vi "MDOAcquire Data from х502 streaming.vi"() -> ()   [LabVIEW 2012]
uses:
  controls/Coeff.ctl
  controls/MDOHW Configuration.ctl
  <vilib>/Analysis/3filter.llb/Filter Passband Type.ctl
  <vilib>/Analysis/3filter.llb/Butterworth Filter (DBL).vi
  <vilib>/Analysis/NI_AALBase.lvlib
panel:
  in  "Hardware Configuration":T1 {"SyncMode" items=["INTERNAL"=0, "EXTERNAL_MASTER"=1, "DI_SYN1_RISE"=2, "DI_SYN1_FALL"=3, "DI_SYN2_RISE"=6, "DI_SYN2_FALL"=7]}
  in  "Coeff":T2={"Coeff_U"=300.0, "Offset_U"=0.0, "Coeff_I"=23.5, "Offset_I"=0.15}
  in  "stop":bool
  out "error out":errorcluster
  in  "error in (no error)":errorcluster
  out "din_data_size":u32
  out "Ток":dbl[](graph)
  out "Напряжение":dbl[](graph)
  out "DIN":u32[](array[numeric]) format="%b"
  in  "IP Addr":string="192.168.0.1"
  out "MCU ver":string
  in  "Отображать за время":dbl=100.0 min=10.0 step=1.0
  out "Установленная частота синхронного ввода DIN":dbl=2.0 min=2.0 max=2000000.0 format="%#_8f"
  in  "Частота синхронного ввода DIN":dbl=20000.0 min=1.0 max=2000000.0 format="%#_8f"
  out "FPGA Ver":string
  out "Установленная частота на канал":dbl=2.0 min=2.0 max=2000000.0 format="%#_8f"
  out "Установленная частота сбора":dbl=2.0 min=2.0 max=2000000.0 format="%#_8f"
  in  "Частота сбора на канал":dbl=50000.0 min=2.0 max=2000000.0 format="%#_8f"
  in  "Частота сбора (Гц)":dbl=100000.0 min=2.0 max=2000000.0 format="%#_8f"
  out "PldaVer":u8
  out "Serial":string
  out "Name":string
  # "Информация о плате"
  # "Настройки модуля"
  # "Устанавливаемое"
  # "Установленное"
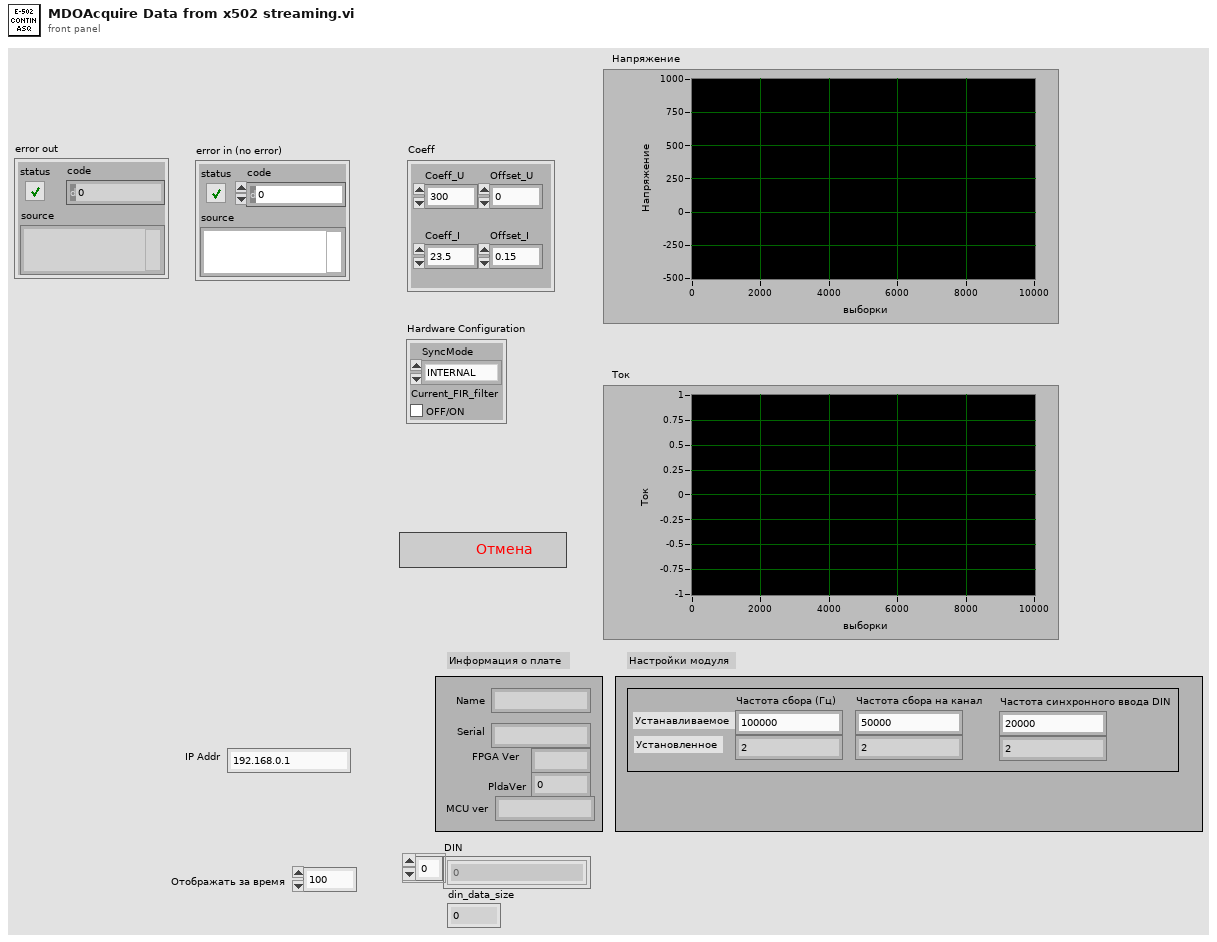
[diagram p1: front panel]
types:
  T1 = typedef "MDOHW Configuration.ctl" = cluster{"SyncMode":u32, "Current_FIR_filter":bool}
  T2 = typedef "Coeff.ctl" = cluster{"Coeff_U":dbl, "Offset_U":dbl, "Coeff_I":dbl, "Offset_I":dbl}
  T3 = cluster{"PhyCh":u32, "Avg":u32, "Mode":u32, "Range":u32}[]
  T4 = typedef "NI_AALBase.lvlib/Filter Passband Type.ctl" = enum32{"Lowpass", "Highpass", "Bandpass", "Bandstop"}
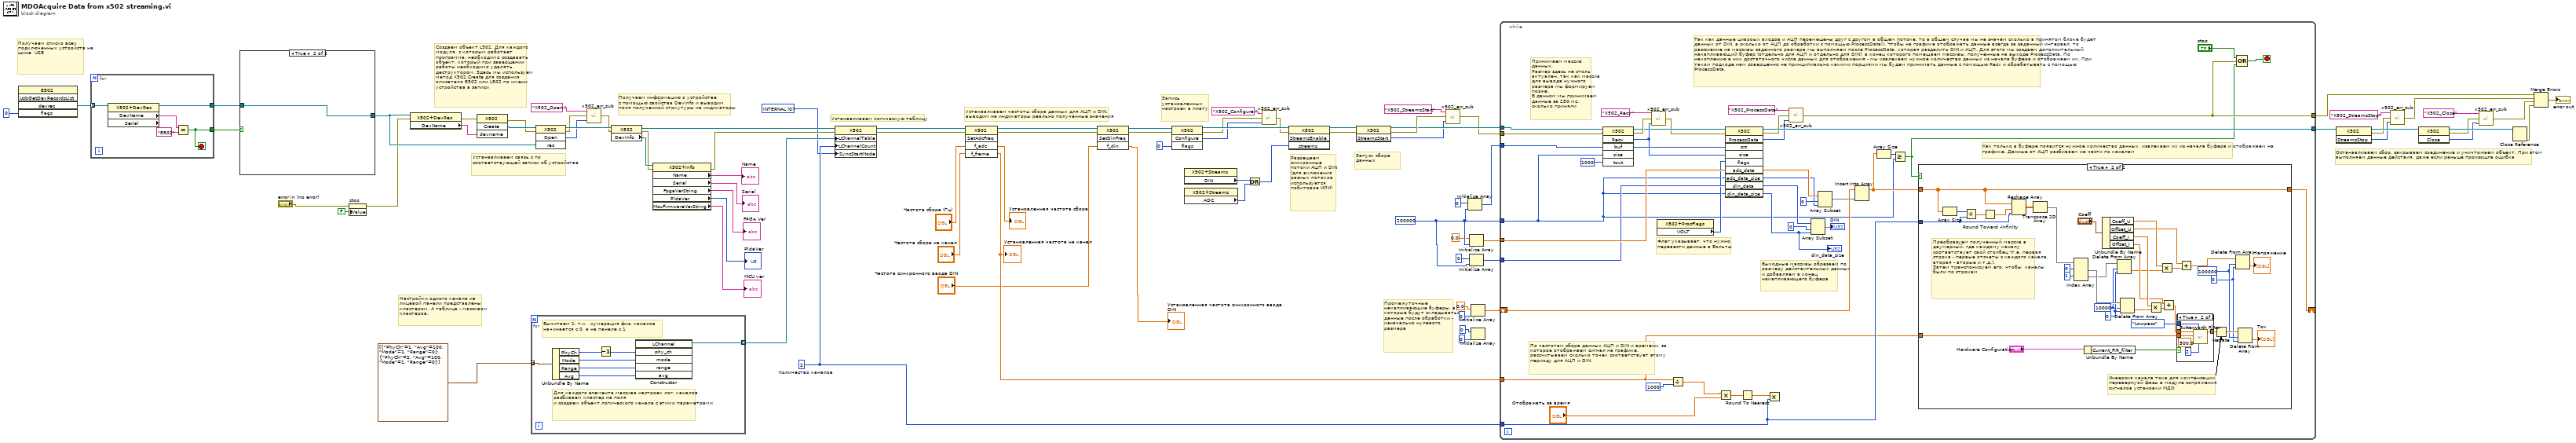
[diagram p0: block diagram]
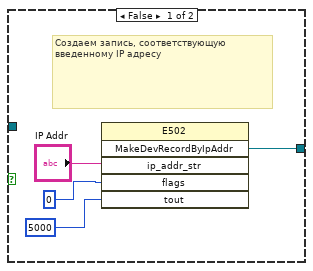
[diagram p4: hidden frame]
diagram:
  w1 = u32 0 items=["INTERNAL"=0, "EXTERNAL_MASTER"=1, "DI_SYN1_RISE"=2, "DI_SYN1_FALL"=3, "DI_SYN2_RISE"=6, "DI_SYN2_FALL"=7] ("SyncStartMode")
  w84 = u32 2  # Количество каналов
  w80 = u32 200000 ("element")
  # "Промежуточные накапливающие буферы, в которые будут складываться данные после обработки - изначально нулевого размера"
  # "Получаем списко всех подключенных устройств на шине  USB"
  # "Останавливаем сбор, закрываем соединение и уничтожаем объект. При этом выполняем данные действия, даже если раньше произошла ошибка"
  # "Запуск сбора данных"
  # "Разрешаем синхронные потоки АЦП и DIN (для включения разных потоков используется побитовое ИЛИ)"
  # "Запись установленных настроек в плату"
  # "Устанавливаем частоты сбора данных для АЦП и DIN,\nвыводим на индикаторы реально полученные значения"
  # "Устанавливаем логическую таблицу"
  # "Настройки одного канала на лицевой панели представлены кластером. А таблица - массивом кластеров."
  # "Создаем объект L502. Для каждого модуля, с которым работает программа, необходимо создавать объект, который при завершении работы необходимо удалять деструктором. Здесь мы используем метод X502.Create для создания описателя E502 или L502 по имени устройства в записи"
  # "Получаем информацию о устройстве \nс помощью свойства DevInfo и выводим\nполя полученной стркутуры на индикаторы"
  # "Устанавливаем связь с по соответствующей записи об устройстве"
  n1 = invoke class="E502" method="UsbGetDevRecordsList"("flags"=0) -> ("devrec"=w14:refnum<k24>[])  [unwired: 4 in, 4 out]
  n2 = for {
    tunnel: w14 -> [w89] mode=indexing
    tunnel: [w88] -> w12
    tunnel: [w85] -> w13
    stop <- w85 stop-if-true
    n3 = property class="X502+DevRec" props=["DevName", "Serial"](reference=w89) -> (reference out=w88:refnum<k24>, "DevName"=w87:string)  [unwired: 1 in, 2 out]
    n4 = Equal?(x=w87, y="E502") -> (x = y?=w85:bool)
  }
  n5 = case shown="True" w13 {
    tunnel: [w90 w94] -> w21
    tunnel: w12 -> [_ w94]
    frame False {
      # "Создаем запись, соответствующую введенному IP адресу"
      n6 = invoke class="E502" method="MakeDevRecordByIpAddr"("ip_addr_str"="IP Addr", "flags"=0, "tout"=5000) -> ("MakeDevRecordByIpAddr"=w90:refnum<k24>)  [unwired: 3 in, 5 out]
    }
    frame True {
    }
  }
  n7 = property on="stop" class="Bool (strict)"(error in="error in (no error)", "Value"=FALSE ("Visible")) -> (error out=w9:errorcluster)  [unwired: 1 in, 1 out]
  n8 = property class="X502+DevRec"(reference=w21, error in=w9) -> (error out=w16:errorcluster, "DevName"=w52:string)  [unwired: 1 out]
  n9 = invoke class="X502" method="Create"(error in=w16, "devname"=w52) -> (error out=w51:errorcluster, "Create"=w53:refnum<k24>)  [unwired: 2 in, 2 out]
  n10 = for {
    tunnel: T3 [{"PhyCh"=1, "Avg"=100, "Mode"=1, "Range"=0}, {"PhyCh"=2, "Avg"=100, "Mode"=1, "Range"=0}] ("Логические каналы") -> [w101] mode=indexing
    tunnel: [w95] -> w76 mode=indexing
    # "Вычитаем 1, т.к.  нумерация физ. каналов начинается с 0, а на панеле с 1"
    # "Для каждого элемента массива настроек лог. каналов разбиваем кластер на поля\nи создаем объект логического канала с этими параметрами"
    n11 = Unbundle By Name(w101) -> ("PhyCh"=w100:u32, "Mode"=w98:u32, "Range"=w97:u32, "Avg"=w96:u32)
    n12 = Decrement(x=w100) -> (x-1=w99:u32)
    n13 = constructor class="X502+LChannel"("phy_ch"=w99, "mode"=w98, "range"=w97, "avg"=w96) -> (reference out=w95:refnum<k24>)  [unwired: 3 in, 6 out]
  }
  n14 = invoke class="X502" method="Open"(reference=w53, error in=w51, "rec"=w21) -> (reference out=w56:refnum<k24>, error out=w49:errorcluster, "Open"=w50:i32)  [unwired: 1 in, 1 out]
  n15 = call "x502_err_sub.vi"("Error code"=w50, "error in (no error)"=w49, "Error descr"="X502_Open ") -> ("error out"=w47:errorcluster)
  n16 = property class="X502"(reference=w56, error in=w47) -> (reference out=w57:refnum<k24>, error out=w45:errorcluster, "DevInfo"=w46:refnum<k24>)
  n17 = property class="X502+Info"(reference=w46, error in=w45) -> (error out=w22:errorcluster, "Name"=→"Name":string, "Serial"=→"Serial":string, "FpgaVerString"=→"FPGA Ver":string, "PldaVer"=→"PldaVer":u8, "McuFirmwareVerString"=→"MCU ver":string)  [unwired: 1 out]
  n18 = property class="X502"(reference=w57, error in=w22, "LChannelTable"=w76, "LChannelCount"=w84, "SyncStartMode"=w1) -> (reference out=w58:refnum<k24>, error out=w59:errorcluster)
  n19 = invoke class="X502" method="SetAdcFreq"(reference=w58, error in=w59, "f_adc"="Частота сбора (Гц)", "f_frame"="Частота сбора на канал") -> (reference out=w63:refnum<k24>, error out=w64:errorcluster, "f_adc"=→"Установленная частота сбора":dbl, "f_frame"=w77:dbl)  [unwired: 1 in, 1 out]
  "Установленная частота на канал" <- w77
  n20 = invoke class="X502" method="SetDinFreq"(reference=w63, error in=w64, "f_din"="Частота синхронного ввода DIN") -> (reference out=w68:refnum<k24>, error out=w69:errorcluster, "f_din"=→"Установленная частота синхронного ввода DIN":dbl)  [unwired: 1 in, 1 out]
  n21 = invoke class="X502" method="Configure"(reference=w68, error in=w69, "flags"=0) -> (reference out=w70:refnum<k24>, error out=w39:errorcluster, "Configure"=w37:i32)  [unwired: 1 in, 1 out]
  n22 = property class="X502+Streams"() -> ("DIN"=w31:u32)  [unwired: 2 in, 2 out]
  n23 = property class="X502+Streams"() -> ("ADC"=w67:u32)  [unwired: 2 in, 2 out]
  n24 = Or(x=w31, y=w67) -> (x .or. y?=w30:u32)
  n25 = call "x502_err_sub.vi"("Error code"=w37, "error in (no error)"=w39, "Error descr"="X502_Configure ") -> ("error out"=w38:errorcluster)
  n26 = invoke class="X502" method="StreamsEnable"(reference=w70, error in=w38, "streams"=w30) -> (reference out=w71:refnum<k24>, error out=w72:errorcluster)  [unwired: 1 in, 2 out]
  n27 = invoke class="X502" method="StreamsStart"(reference=w71, error in=w72) -> (reference out=w33:refnum<k24>, error out=w35:errorcluster, "StreamsStart"=w7:i32)  [unwired: 1 in]
  n28 = call "x502_err_sub.vi"("Error code"=w7, "error in (no error)"=w35, "Error descr"="X502_StreamsStart") -> ("error out"=w32:errorcluster)
  n29 = Initialize Array(u32 0 ("element"), w80) -> (w81:u32[])
  n30 = Initialize Array(0.0 ("element"), w80) -> (w83:dbl[])
  n31 = Initialize Array(u32 0 ("element"), w80) -> (w82:u32[])
  n32 = Initialize Array(0.0 ("element"), u32 0 ("element")) -> (w2:dbl[])
  n33 = Initialize Array(u32 0 ("element"), u32 0 ("element")) -> ()  [unwired: 1 out]
  n34 = while {
    tunnel: w84 -> [w142]
    tunnel: w83 -> [w141]
    tunnel: w82 -> [w140]
    tunnel: w81 -> [w139]
    tunnel: w80 -> [w103]
    tunnel: w77 -> [w112]
    tunnel: w33 -> [w138]
    tunnel: w32 -> [w137]
    tunnel: [w136] -> w29
    tunnel: [w114] -> w17
    shift-right: [w106] -> _
    shift-left: w2 -> [w107]
    stop <- w113 stop-if-true
    # "Так как данные цивроых входов и АЦП перемешены друг с другом в общем потоке, то в общем случае мы не значем сколько в принятом блоке будет данных от DIN, а сколько от АЦП до обработки с помощью ProcessData(). Чтобы на графике отображать данные всегда за заданный интервал, то разюиение на массивы заданного размера мы выполняем после ProcessData, которая разделить DIN и АЦП. Для этого мы создаем дополнительный накапливающий буфер (отдельно для АЦП и отдельно для DIN), в конец которого помещаем массивы, полученные на выходе ProcessData. По накоплению в них достаточного числа данных для отображения - мы извлекаем нужное количество данных из начала буфера и отображаем их. При таком подходе нам совершенно не принципиально какими порциями мы будем принимать данные с помощью Recv и обрабатывать с помощью ProcessData."
    # "Как только в буфере появится нужное количество данных, извлекаем их из начала буфера и отображаем на графике. Данные от АЦП разбиваем на части по каналам"
    # "По частотам сбора данных АЦП и DIN и времени, за которое отображаем сигнал на графике, рассчитываем сколько точек соответствует этому периоду для АЦП и DIN."
    # "Выходные массивы обрезаем по размеру действительных данных и добавляем в конец накапливающего буфера"
    # "Флаг указывает, что нужно перевести данные в Вольты"
    # "Принимаем массив данных.\nРазмер здесь не столь актуален, так как массив для вывода нужного размера мы формируем позже.\nВ данном мы принимаем данные за 250 мс, сколько приняли"
    n35 = invoke class="X502" method="Recv"(reference=w138, error in=w137, "buf"=w139, "size"=w103, "tout"=u32 1000 ("element")) -> (reference out=w117:refnum<k24>, error out=w123:errorcluster, "Recv"=w122:i32, "buf"=w135:u32[])  [unwired: 1 in, 2 out]
    n36 = call "x502_err_sub.vi"("Error code"=w122, "error in (no error)"=w123, "Error descr"="X502_Recv") -> ("error out"=w116:errorcluster)
    n37 = property class="X502+ProcFlags"() -> ("VOLT"=w133:u32)  [unwired: 2 in, 2 out]
    n38 = Divide(x=w112, y=1000) -> (x/y=w128:dbl)
    n39 = Multiply(x=w128, y="Отображать за время") -> (x*y=w127:dbl)
    n40 = invoke class="X502" method="ProcessData"(reference=w117, error in=w116, "src"=w135, "size"=w122, "flags"=w133, "adc_data"=w141, "adc_data_size"=w103, "din_data"=w140, "din_data_size"=w103) -> (reference out=w136:refnum<k24>, error out=w120:errorcluster, "ProcessData"=w119:i32, "adc_data"=w111:dbl[], "adc_data_size"=w109:u32, "din_data"=w131:u32[], "din_data_size"=w130:u32)  [unwired: 1 in, 3 out]
    "din_data_size" <- w130
    n41 = Round To Nearest(number=w127) -> (nearest integer value=w126:dbl)
    n42 = Multiply(x=w126, y=w142) -> ()  [unwired: 1 out]
    n43 = call "x502_err_sub.vi"("Error code"=w119, "error in (no error)"=w120, "Error descr"="X502_ProcessData") -> ("error out"=w114:errorcluster)
    n44 = Array Subset(array=w131, index=u32 0 ("element"), length=w130) -> (→"DIN":u32[])
    n45 = Array Subset(array=w111, index=0, length=w109) -> (w108:dbl[])
    n46 = Insert Into Array(array=w107, new element=w108) -> (w105:dbl[])  [unwired: 1 in]
    n47 = Array Size(array=w105) -> (size(s)=w104:i32)
    n48 = Greater Or Equal?(x=w104, y=w103) -> (x >= y?=w102:bool)
    n49 = case shown="True" w102 {
      tunnel: w142 -> [_ w177]
      tunnel: w112 -> [_ w169]
      tunnel: w105 -> [w143 w146]
      tunnel: [w143 w146] -> w106
      frame False {
      }
      frame True {
        w148 = 0 ("index")
        w149 = 100000 ("length")
        w155 = 0 ("index")
        w154 = 10000 ("length")
        # "Инверсия канала тока для компенсации \nперевернуой фазы в модуле сопряжения \nсигналов установки МДО"
        # "Преобразуем полученный массив в двумерный, где каждому каналу соответствует свой столбец (т.е. первая строка - первые отсчеты с каждого канала, вторая - вторые и т.д.).\nЗатем транспонируем его, чтобы  каналы были по строкам"
        n50 = Array Size(array=w146) -> (size(s)=w147:i32)
        n51 = Divide(x=w147, y=w177) -> (x/y=w176:dbl)
        n52 = Round Toward -Infinity(1:w176) -> (0:w175:dbl)
        n53 = Reshape Array(w146, w175, w177) -> (w170:dbl[][])
        n54 = Transpose 2D Array(2D array=w170) -> (transposed array=w160:dbl[][])
        n55 = Index Array(array=w160, index (row) #1=0 ("index (row)"), index (row) #2=1 ("index (row)")) -> (element #1=w159:dbl[], element #2=w156:dbl[])  [unwired: 2 in]
        n56 = Unbundle By Name("Hardware Configuration") -> ("Current_FIR_filter"=w145:bool)
        n57 = Unbundle By Name("Coeff") -> ("Coeff_U"=w163:dbl, "Offset_U"=w164:dbl, "Coeff_I"=w162:dbl, "Offset_I"=w161:dbl)
        n58 = Delete From Array(array=w156, length=w154, index=w155) -> (deleted portion=w157:dbl[])  [unwired: 1 out]
        n59 = Delete From Array(array=w159, length=w154, index=w155) -> (deleted portion=w158:dbl[])  [unwired: 1 out]
        n60 = Multiply(x=w162, y=w158) -> (x*y=w172:dbl[])
        n61 = Multiply(x=w163, y=w157) -> (x*y=w171:dbl[])
        n62 = Add(x=w161, y=w172) -> (x+y=w167:dbl[])
        n63 = case shown="True" w145 {
          tunnel: w169 -> [_ w184]
          tunnel: Filter_Passband_Type."Lowpass" ("filter type") -> [_ w183]
          tunnel: w167 -> [w178 w181]
          tunnel: [w178 w179] -> w166
          frame False {
          }
          frame True {
            n64 = call-poly <vilib>:"Butterworth Filter.vi"("order"=2, "filter type"=w183, "low cutoff freq: fl"=500.0, "sampling freq: fs"=w184, "X"=w181) -> ("Filtered X"=w179:dbl[])  [unwired: 3 in, 1 out]
          }
        }
        n65 = Add(x=w164, y=w171) -> (x+y=w153:dbl[])
        n66 = Negate(x=w166) -> (-x=w151:dbl[])
        n67 = Delete From Array(array=w153, length=w149, index=w148) -> (deleted portion=→"Напряжение":dbl[])  [unwired: 1 out]
        n68 = Delete From Array(array=w151, length=w149, index=w148) -> (deleted portion=→"Ток":dbl[])  [unwired: 1 out]
      }
    }
    n69 = Compound Arithmetic op=OR("stop", w114, w102) -> (w113:bool)
  }
  n70 = invoke class="X502" method="StreamsStop"(reference=w29) -> (reference out=w54:refnum<k24>, error out=w28:errorcluster, "StreamsStop"=w26:i32)  [unwired: 2 in]
  n71 = call "x502_err_sub.vi"("Error code"=w26, "error in (no error)"=w28, "Error descr"="X502_StreamsStop") -> ("error out"=w18:errorcluster)
  n72 = invoke class="X502" method="Close"(reference=w54) -> (reference out=w55:refnum<k24>, error out=w24:errorcluster, "Close"=w23:i32)  [unwired: 2 in]
  n73 = call "x502_err_sub.vi"("Error code"=w23, "error in (no error)"=w24, "Error descr"="X502_Close") -> ("error out"=w19:errorcluster)
  n74 = Close Reference(reference=w55) -> (error out=w20:errorcluster)  [unwired: 1 in]
  n75 = Merge Errors(w17, w18, w19, w20) -> (→"error out":errorcluster)
